vi "OPEN USER OR ITEM.vi"(9 "USER OR ITEM":enum16{"USER", "ITEM"}(ring), 10 "DATA IN":string[][](array[string]), 11 "REFERENCES":T1) -> (2 "INVALID INPUT":bool, 3 "USER/ITEM DATA TRANSFER":T2(array[cluster]))   [LabVIEW 2019]
uses:
  Controls/References Cluster.ctl
  <vilib>/userDefined/High Color/IMAQdx.ctl
  Controls/Custom Calendar/Custom Calendar.xctl
  Controls/Column Enums/Inventory Column Enum.ctl
  Controls/Column Enums/User Column Enum.ctl
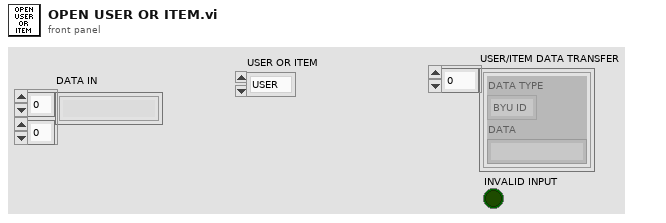
[diagram p1: front panel]
types:
  T1 = typedef "References Cluster.ctl" = cluster{"MAIN PAGES":refnum<vi>, "ADD/EDIT ITEM REFERENCES":cluster{"Identifier":refnum<vi>, "BYU ICN #":refnum<vi>, "Item Description":refnum<vi>, "Comments":refnum<vi>, "Checked Out Date":refnum<vi>, "Due Date":refnum<vi>, "Check Out Location":refnum<vi>, "Reminder Count":refnum<vi>, "Most Recent Reminder Date":refnum<vi>, "BYU ID #":refnum<vi>, "Building/Room":refnum<vi>, "Location in Room":refnum<vi>, "Manual":refnum<vi>, "Manufacturer":refnum<vi>, "Model #":refnum<vi>, "Serial #":refnum<vi>, "Date Acquired":refnum<vi>, "ADD/EDIT ITEM LABEL":refnum<vi>, "ARCHIVE ITEM":refnum<vi>, "Archive Item Inputs":refnum<vi>, "Reminder Notes":refnum<vi>, "DUPLICATE ITEM":refnum<vi>}, "ADD/EDIT USER REFERENCES":cluster{"BYU ID # (##-###-####)":refnum<vi>, "First Name":refnum<vi>, "Last Name":refnum<vi>, "Phone Number (###-###-####)":refnum<vi>, "Email":refnum<vi>, "Department":refnum<vi>, "Graduation Status":refnum<vi>, "Anticipated Graduation Year":refnum<vi>, "Credit Score":refnum<vi>, "Date Added":refnum<vi>, "Graduation Clearance Date":refnum<vi>, "Picture File Name":refnum<vi>, "ADD/EDIT USER LABEL":refnum<vi>, "Department Map":refnum<vi>, "Status Map":refnum<vi>, "Anticipated Graduation Year Map":refnum<vi>, "User Agreement":refnum<vi>, "User Comments":refnum<vi>, "Camera":refnum<vi>}, "RETURN ITEM REFERENCES":cluster{"Item or Person:":refnum<vi>, "Search Return Results":refnum<vi>, "What are you searching for?":refnum<vi>}, "SEARCH DATABASE REFERENCES":cluster{"What to Search For:":refnum<vi>, "Where to Search":refnum<vi>, "Column to Search In":refnum<vi>, "Column to Sort By":refnum<vi>, "Search Database Results":refnum<vi>, "Inventory Column Selector":refnum<vi>, "User Column Selector":refnum<vi>, "Inventory Archive Column Selector":refnum<vi>, "User Archive Column Selector":refnum<vi>, "Sales Tracking Column Selector":refnum<vi>, "Checked In Archive Column Selector":refnum<vi>, "Restore User":refnum<vi>, "Date Range":refnum<vi>, "Dates Less Than":refnum<vi>, "Dates Greater Than":refnum<vi>, "Search Print Receipt":refnum<vi>, "Edit Sale Description":refnum<vi>}, "USER ITEMS REFERENCES":cluster{"USER'S INFORMATION":refnum<vi>, "User's Checked Out Items":refnum<vi>, "User Info Comments":refnum<vi>, "SEE USER INFO COMMENTS":refnum<vi>}, "EDIT ITEMS REFERENCES":cluster{"New Check Out Location":refnum<vi>, "Items to Edit":refnum<vi>, "Edit Items Due Date":refnum<vi>, "New Reminder Notes":refnum<vi>, "New Item Description":refnum<vi>}, "CHECK OUT ITEMS REFERENCES":cluster{"Enter Item:":refnum<vi>, "Check Out Items Due Date":refnum<vi>, "Check Out Location":refnum<vi>, "Items to be Checked Out":refnum<vi>, "Possible Items":refnum<vi>, "Altered Item Description":refnum<vi>}, "TRANSFER ITEMS REFERENCES":cluster{"Search Parameter":refnum<vi>, "What to Match":refnum<vi>, "Matching Individuals":refnum<vi>, "Items to be Transferred":refnum<vi>}, "SETTINGS REFERENCES":cluster{"PSC Database Settings":refnum<vi>, "PSC Sales Item Spreadsheet":refnum<vi>}, "PSC SALES REFERENCES":cluster{"BYU ID CARD #":refnum<vi>, "Sale Description":refnum<vi>, "Scan or Enter Item Name":refnum<vi>, "Items to be Sold":refnum<vi>, "Grand Total":refnum<vi>, "Item List":refnum<vi>}}
  T2 = cluster{"DATA TYPE":enum16{"BYU ID", "ME#/IDENTIFIER", "BYU ICN"}, "DATA":string}[]
  T3 = cluster{"DATA TYPE":enum16{"BYU ID", "ME#/IDENTIFIER", "BYU ICN"}, "DATA":string}
  T4 = cluster{"What to Search For:":refnum<vi>, "Where to Search":refnum<vi>, "Column to Search In":refnum<vi>, "Column to Sort By":refnum<vi>, "Search Database Results":refnum<vi>, "Inventory Column Selector":refnum<vi>, "User Column Selector":refnum<vi>, "Inventory Archive Column Selector":refnum<vi>, "User Archive Column Selector":refnum<vi>, "Sales Tracking Column Selector":refnum<vi>, "Checked In Archive Column Selector":refnum<vi>, "Restore User":refnum<vi>, "Date Range":refnum<vi>, "Dates Less Than":refnum<vi>, "Dates Greater Than":refnum<vi>, "Search Print Receipt":refnum<vi>, "Edit Sale Description":refnum<vi>}
  T5 = typedef "Inventory Column Enum.ctl" = enum16{"Identifier", "BYU ICN #", "Item Description", "Comments", "Checked Out Date", "Due Date", "Check Out Location", "Reminder Count", "Most Recent Reminder Date", "BYU ID #", "Building/Room", "Location in Room", "Manual", "Manufacturer", "Model #", "Serial #", "Date Acquired"}
  T6 = typedef "User Column Enum.ctl" = enum16{"BYU ID #", "First Name", "Last Name", "Phone Number", "Email", "Department", "Graduation Status", "Anticipated Graduation Year", "Credit Score", "Date Added", "Graduation Clearance Date", "Picture File Name"}
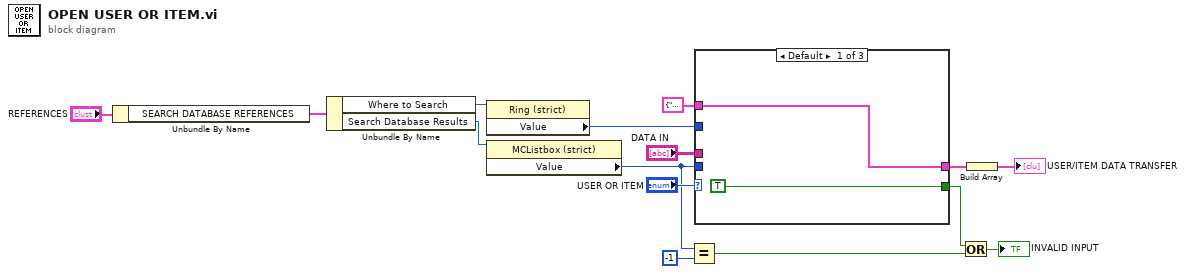
[diagram p0: block diagram]
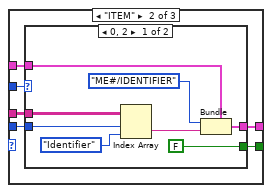
[diagram p2: hidden frame]
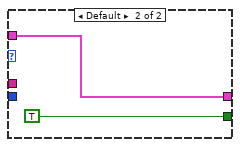
[diagram p3: hidden frame]
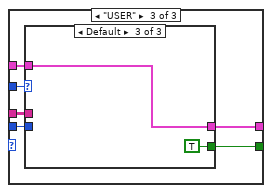
[diagram p4: hidden frame]
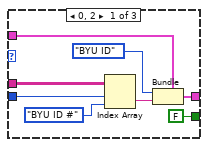
[diagram p5: hidden frame]
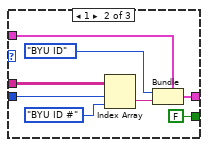
[diagram p6: hidden frame]
diagram:
  n1 = Unbundle By Name("REFERENCES") -> ("SEARCH DATABASE REFERENCES"=w6:T4)
  n2 = Unbundle By Name(w6) -> ("Where to Search"=w15:refnum<vi>, "Search Database Results"=w13:refnum<vi>)
  n3 = property class="Ring (strict)"(reference=w15) -> ("Value"=w14:u16)  [unwired: 1 in, 2 out]
  n4 = property class="MCListbox (strict)"(reference=w13) -> ("Value"=w5:i32)  [unwired: 1 in, 2 out]
  n5 = Equal?(x=w5, y=-1) -> (x = y?=w2:bool)
  n6 = case shown="Default" "USER OR ITEM" {
    tunnel: w14 -> [_ w23 w39]
    tunnel: "DATA IN" -> [_ w22 w38]
    tunnel: w5 -> [_ w21 w37]
    tunnel: T3 {"DATA TYPE"=enum."BYU ID", "DATA"=""} ("USER/ITEM DATA TRANSFER") -> [w17 w20 w36]
    tunnel: [w17 w19 w35] -> w9
    tunnel: [TRUE ("x") w18 w34] -> w1
    frame Default {
    }
    frame "ITEM" {
      n7 = case shown="0, 2" w23 {
        tunnel: w22 -> [w30 _]
        tunnel: w21 -> [w29 _]
        tunnel: w20 -> [w31 w33]
        tunnel: [w28 w33] -> w19
        tunnel: [FALSE ("x") TRUE ("x")] -> w18
        frame 0, 2 {
          n8 = Index Array(array=w30, index (row)=w29, index (col)=Inventory_Column_Enum."Identifier" ("INVENTORY COLUMN ENUM")) -> (element=w26:string)
          n9 = Bundle(cluster=w31, "DATA TYPE"=enum16{"BYU ID", "ME#/IDENTIFIER", "BYU ICN"}."ME#/IDENTIFIER", "DATA"=w26) -> (w28:T3)
        }
        frame Default {
        }
      }
    }
    frame "USER" {
      n10 = case shown="Default" w39 {
        tunnel: w38 -> [w46 w54 _]
        tunnel: w37 -> [w44 w52 _]
        tunnel: w36 -> [w47 w55 w57]
        tunnel: [w43 w51 w57] -> w35
        tunnel: [FALSE ("x") FALSE ("x") TRUE ("x")] -> w34
        frame 0, 2 {
          n11 = Index Array(array=w46, index (row)=w44, index (col)=Inventory_Column_Enum."BYU ID #" ("INVENTORY COLUMN ENUM")) -> (element=w42:string)
          n12 = Bundle(cluster=w47, "DATA TYPE"=enum16{"BYU ID", "ME#/IDENTIFIER", "BYU ICN"}."BYU ID", "DATA"=w42) -> (w43:T3)
        }
        frame 1 {
          n13 = Index Array(array=w54, index (row)=w52, index (col)=User_Column_Enum."BYU ID #" ("USER COLUMN ENUM")) -> (element=w50:string)
          n14 = Bundle(cluster=w55, "DATA TYPE"=enum16{"BYU ID", "ME#/IDENTIFIER", "BYU ICN"}."BYU ID", "DATA"=w50) -> (w51:T3)
        }
        frame Default {
        }
      }
    }
  }
  n15 = Or(x=w1, y=w2) -> (x .or. y?=→"INVALID INPUT":bool)
  n16 = Build Array(w9) -> (→"USER/ITEM DATA TRANSFER":T2)
